vi "OM_FromLabVIEW.vi"(8 "error in (no error)":errorcluster, 11 "Vehicle2 in":refnum<class "Vehicle2.lvclass">) -> (0 "error out":errorcluster, 2 "DbRow":variant, 3 "Vehicle2 out":refnum<class "Vehicle2.lvclass">)   [LabVIEW 2020, in "ORM_Examples.lvlib" / "Vehicle2.lvclass"]
uses:
  Vehicle2.lvclass
  Vehicle2.lvclass/Vehicle2.ctl
  Read Make.vi
  Read Model.vi
  Read Year.vi
  Read VehicleID.vi
  <vilib>/JDP Science/JSONtext/JSONtext.lvlib
panel:
  out "<JSON>":string
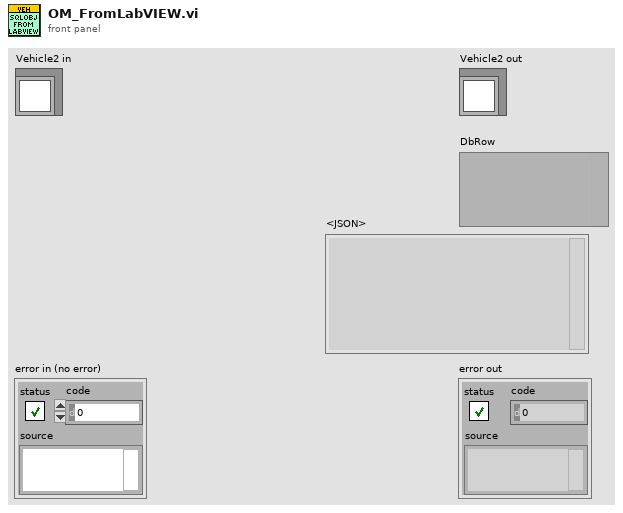
[diagram p1: front panel]
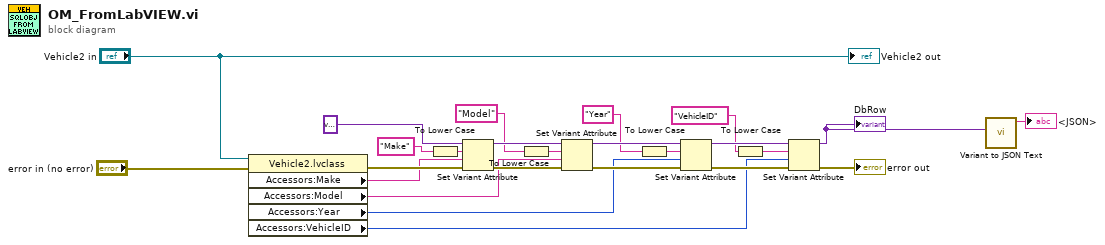
[diagram p0: block diagram]
diagram:
  n1 = property class="Vehicle2.lvclass"(reference="Vehicle2 in", error in="error in (no error)") -> (error out=w25:errorcluster, "Accessors:Make"=w19:string, "Accessors:Model"=w18:string, "Accessors:Year"=w17:i32, "Accessors:VehicleID"=w14:i32)  [unwired: 1 out]
  n2 = To Lower Case(string="Make" ("name")) -> (all lower case string=w10:string)
  n3 = Set Variant Attribute(Variant=variant, name=w10, value=w19, error in=w25) -> (Variant out=w23:variant, error out=w22:errorcluster)  [unwired: 1 out]
  n4 = To Lower Case(string="Model" ("name")) -> (all lower case string=w9:string)
  n5 = Set Variant Attribute(Variant=w23, name=w9, value=w18, error in=w22) -> (Variant out=w21:variant, error out=w20:errorcluster)  [unwired: 1 out]
  n6 = To Lower Case(string="Year" ("name")) -> (all lower case string=w8:string)
  n7 = Set Variant Attribute(Variant=w21, name=w8, value=w17, error in=w20) -> (Variant out=w15:variant, error out=w16:errorcluster)  [unwired: 1 out]
  n8 = To Lower Case(string="VehicleID" ("name")) -> (all lower case string=w7:string)
  n9 = Set Variant Attribute(Variant=w15, name=w7, value=w14, error in=w16) -> (Variant out=w2:variant, error out=→"error out":errorcluster)  [unwired: 1 out]
  "DbRow" <- w2
  n10 = call <vilib>:"Variant to JSON Text.vi"("Variant"=w2) -> ("<JSON>"=→"<JSON>":string)  [unwired: 8 in, 2 out]
  "Vehicle2 out" <- "Vehicle2 in"
